vi "SYST_PREF_ITEM_RETR_POW.vi"(0 "VISA IN":refnum<visa-resource-name>, 5 "error in":errorcluster, 7 "Power":bool) -> (14 "VISA Out":refnum<visa-resource-name>, 19 "error out":errorcluster)   [LabVIEW 2018, in "PNA-X.lvlib"]
doc: "SYSTem:PREFerences:ITEM:RETRace:POWer <char> \n1878\n\n(Read-Write) For single-band frequency or segment sweeps ONLY, specify whether to turn RF power \nON or OFF during a retrace. Learn more about RF power during sweep retrace. \nTo send this command using the PNA front panel, open the GPIB Command Processor Console, then \ntype either of the following examples at the command prompt. Then type the Query Syntax and press \nenter to be sure the PNA took the command. \nThis setting remains until changed using this command, or until the hard drive is changed or \nreformatted. \nParameters \n<char> Choose from: \nAUTO: Power is left ON during retrace of single-band frequency or segment \nsweeps ONLY. \nOFF: Power is turned OFF during retrace of single-band frequency or segment \nsweeps ONLY. \nExamples SYST:PREF:ITEM:RETR:POW OFF \nsystem:preferences:item:retrace:power auto \nQuery Syntax SYSTem:PREFerences:ITEM:RETRace:POWer? \nReturn Type Character \nDefault AUTO"
uses:
  PNA-X.lvlib
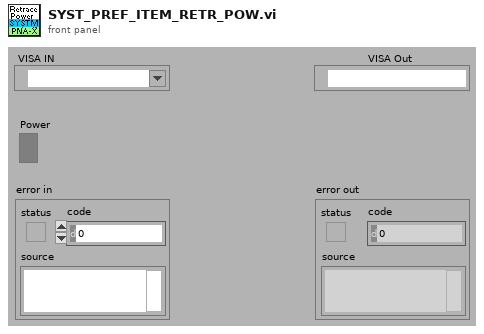
[diagram p1: front panel]
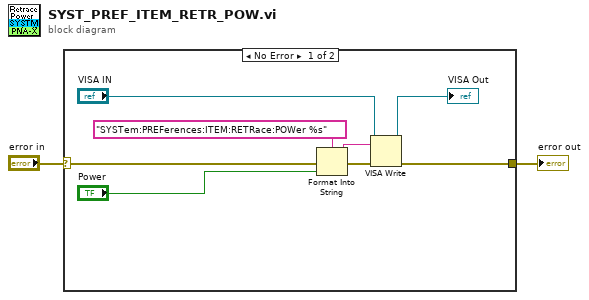
[diagram p0: block diagram]
diagram:
  n1 = case shown="No Error" "error in" {
    selector: "error in" -> [w10 w11]
    tunnel: [w5 w11] -> w1
    frame No Error {
      n2 = Format Into String(format string="SYSTem:PREFerences:ITEM:RETRace:POWer %s" ("Cmdline"), error in=w10, "Power") -> (resulting string=w8:string, error out=w9:errorcluster)  [unwired: 1 in]
      n3 = VISA Write(VISA resource name="VISA IN", write buffer=w8, error in (no error)=w9) -> (VISA resource name out=→"VISA Out":refnum<visa-resource-name>, error out=w5:errorcluster)  [unwired: 1 out]
    }
    frame Error {
    }
  }
  "error out" <- w1
